vi "Configure Analog Output.vi"(8 "error in (no error)":errorcluster, 9 "characteristic":u16(ring) items=["log", "log a", "log -6", "log -3", "log +0", "log +3", "log c1", "log c2", "log c3", "lin -10", "lin -9", "lin -8", "lin -7", "lin -6", "lin -5", "lin -4", "lin -3", "lin -2", "lin -1", "lin +0", "lin +1", "lin +2", "lin +3", "IM221", "log c4", "PM411", "ch x", "PRM10K", "IMR110", "IMR120", "IMR310", "IMR320"], 10 "channel":u16(ring) items=["channel 1", "channel 2", "channel 3"], 11 "VGC in":refnum<class "PL Inficon VGC.lvclass">) -> (0 "error out":errorcluster, 1 "characteristic":u16(ring) items=["log", "log a", "log -6", "log -3", "log +0", "log +3", "log c1", "log c2", "log c3", "lin -10", "lin -9", "lin -8", "lin -7", "lin -6", "lin -5", "lin -4", "lin -3", "lin -2", "lin -1", "lin +0", "lin +1", "lin +2", "lin +3", "IM221", "log c4", "PM411", "ch x", "PRM10K", "IMR110", "IMR120", "IMR310", "IMR320"], 2 "channel":u16(ring) items=["channel 1", "channel 2", "channel 3"], 3 "VGC out":refnum<class "PL Inficon VGC.lvclass">)   [LabVIEW 2015, in "PL Inficon VGC.lvclass"]
doc: "Configures analog output."
uses:
  PL Inficon VGC.lvclass
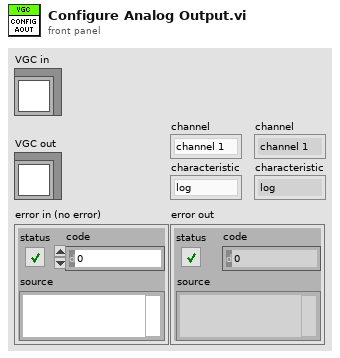
[diagram p1: front panel]
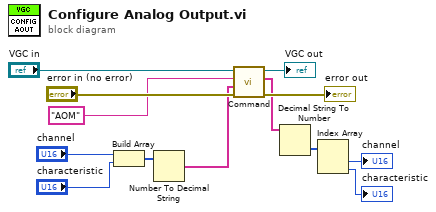
[diagram p0: block diagram]
diagram:
  n1 = Build Array("channel", "characteristic") -> (w7:u16[])
  n2 = Number To Decimal String(number=w7) -> (decimal integer string=w1:string[])  [unwired: 1 in]
  n3 = call "Command.vi"("error in (no error)"="error in (no error)", "parameters"=w1, "command"="AOM" ("format string"), "VGC in"="VGC in") -> ("error out"=→"error out":errorcluster, "response data"=w5:string[], "VGC out"=→"VGC out":refnum<class "PL Inficon VGC.lvclass">)  [unwired: 5 in]
  n4 = Decimal String To Number(string=w5) -> (number=w8:i32[])  [unwired: 2 in, 1 out]
  n5 = Index Array(array=w8) -> (element #1=→"channel":i32, element #2=→"characteristic":i32)  [unwired: 2 in]
